vi "Launch Transfer Line.vi"(8 "error in (no error)":errorcluster, 11 "cRIO-CO2 in":refnum<class "cRIO-CO2.lvclass">) -> (0 "error out":errorcluster, 3 "cRIO-CO2 out":refnum<class "cRIO-CO2.lvclass">)   [LabVIEW 2015, in "cRIO-Carbondioxide.lvlib" / "cRIO-CO2.lvlib" / "cRIO-CO2.lvclass"]
uses:
  cRIO-CO2.lvclass
  CO2 Actor/CO2 Actor.lvclass
  Transfer Line/Transfer Line.lvclass
  <vilib>/ActorFramework/Actor/Actor.lvclass
  cRIO-CO2.lvclass/cRIO-CO2.ctl
  Transfer Line/Transfer Line.lvclass/Transfer Line.ctl
  cRIO-CO2 Messages/Log Message Msg/Log Message Msg.lvclass/Log Message Msg.ctl
  <vilib>/ActorFramework/Message Enqueuer/Message Enqueuer.lvclass/Message Enqueuer.ctl
  <vilib>/ActorFramework/Message Enqueuer/Enqueue.vi
  <vilib>/ActorFramework/Message Priority Queue/Priority Enqueue.vi
  <vilib>/ActorFramework/Message Enqueuer/Message Enqueuer.lvclass
  cRIO-CO2 Messages/Log Message Msg/Log Message Msg.lvclass
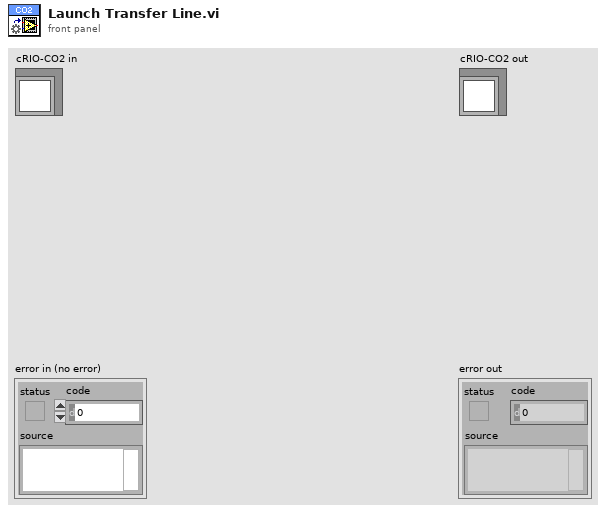
[diagram p1: front panel]
types:
  T1 = typedef "Dedicated Enqueuers.ctl" = cluster{"Freezers":cluster{"Syringe":refnum<class "Message Enqueuer.lvclass">, "Tank 1":refnum<class "Message Enqueuer.lvclass">, "Tank 2":refnum<class "Message Enqueuer.lvclass">, "Tank 3":refnum<class "Message Enqueuer.lvclass">, "Tank 4":refnum<class "Message Enqueuer.lvclass">}, "Heaters":cluster{"Syringe":refnum<class "Message Enqueuer.lvclass">, "Piston":refnum<class "Message Enqueuer.lvclass">}, "Blowers":cluster{"Tank 1":refnum<class "Message Enqueuer.lvclass">, "Tank 2":refnum<class "Message Enqueuer.lvclass">, "Tank 3":refnum<class "Message Enqueuer.lvclass">, "Tank 4":refnum<class "Message Enqueuer.lvclass">, "Syringe":refnum<class "Message Enqueuer.lvclass">}, "Sample Line":refnum<class "Message Enqueuer.lvclass">, "Storage Line":refnum<class "Message Enqueuer.lvclass">, "Transfer Line":refnum<class "Message Enqueuer.lvclass">, "Syringe Stepper":refnum<class "Message Enqueuer.lvclass">, "Syringe Line":refnum<class "Message Enqueuer.lvclass">, "Capillary Line":refnum<class "Message Enqueuer.lvclass">, "Preparation Line":refnum<class "Message Enqueuer.lvclass">, "Turbo":refnum<class "Message Enqueuer.lvclass">, "Vacuum":refnum<class "Message Enqueuer.lvclass">, "He Line":refnum<class "Message Enqueuer.lvclass">, "Cylinder":refnum<class "Message Enqueuer.lvclass">}
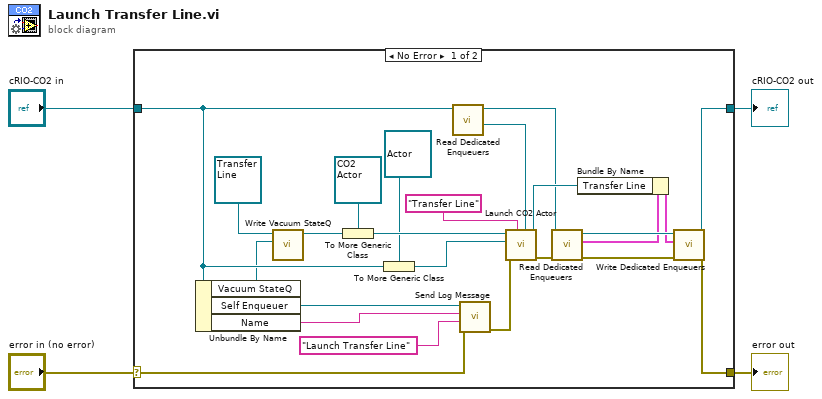
[diagram p0: block diagram]
diagram:
  n1 = case shown="No Error" "error in (no error)" {
    selector: "error in (no error)" -> [w25 w30]
    tunnel: [w16 w30] -> w3
    tunnel: [w13 w29] -> w1
    tunnel: "cRIO-CO2 in" -> [w10 w29]
    frame No Error {
      n2 = Unbundle By Name(w10) -> ("Vacuum StateQ"=w5:refnum<queue>, "Self Enqueuer"=w20:refnum<class "Message Enqueuer.lvclass">, "Name"=w22:string)
      n3 = call "Write Vacuum StateQ.vi"("Vacuum StateQ"=w5, "Transfer Line in"=refnum<class "Transfer Line.lvclass"> refnum ("Transfer Line.lvclass")) -> ("Transfer Line out"=w6:refnum<class "Transfer Line.lvclass">)  [unwired: 9 in]
      n4 = To More Generic Class(target class=refnum<class "CO2 Actor.lvclass"> refnum ("CO2 Actor in"), reference=w6) -> (generic class reference=w28:refnum<class "CO2 Actor.lvclass">)
      n5 = To More Generic Class(target class=refnum<class "Actor.lvclass"> refnum ("Caller Actor in"), reference=w10) -> (generic class reference=w11:refnum<class "Actor.lvclass">)
      n6 = call "Read Dedicated Enqueuers.vi"("cRIO-CO2 in"=w10) -> ("Qs.DedicatedEnQrs"=w8:refnum<queue>, "cRIO-CO2 out"=w9:refnum<class "cRIO-CO2.lvclass">)  [unwired: 7 in, 2 out]
      n7 = call "Send Log Message.vi"("error in (no error)"=w25, "String"="Launch Transfer Line", "Source Name"=w22, "Message Enqueuer"=w20) -> ("error out"=w24:errorcluster)  [unwired: 6 in, 1 out]
      n8 = call "Launch CO2 Actor.vi"("DedicatedEnQrs"=w8, "Name"="Transfer Line", "error in (no error)"=w24, "Caller Actor in"=w11, "CO2 Actor in"=w28) -> ("error out"=w17:errorcluster, "Caller-To-Actor Enqueuer"=w26:refnum<class "Message Enqueuer.lvclass">)  [unwired: 5 in]
      n9 = call "Read Dedicated Enqueuers.vi"("error in (no error)"=w17, "cRIO-CO2 in"=w9) -> ("error out"=w19:errorcluster, "Dedicated Enqueuers"=w15:T1, "cRIO-CO2 out"=w18:refnum<class "cRIO-CO2.lvclass">)  [unwired: 6 in, 1 out]
      n10 = Bundle By Name(cluster=w15, "Transfer Line"=w26) -> (w14:T1)
      n11 = call "Write Dedicated Enqueuers.vi"("error in (no error)"=w19, "Dedicated Enqueuers"=w14, "cRIO-CO2 in"=w18) -> ("error out"=w16:errorcluster, "cRIO-CO2 out"=w13:refnum<class "cRIO-CO2.lvclass">)  [unwired: 7 in]
    }
    frame Error {
    }
  }
  "error out" <- w3
  "cRIO-CO2 out" <- w1
